vi "selectSurroundingPlatforms.vi"(9 "Number of surrounding\nplatforms to raise":i32=2, 11 "Start platform":i32) -> (2 "Platforms \nto raise":i32[](array[numeric]))   [LabVIEW 2017]
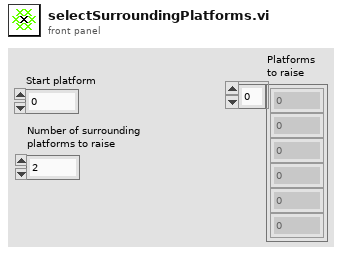
[diagram p1: front panel]
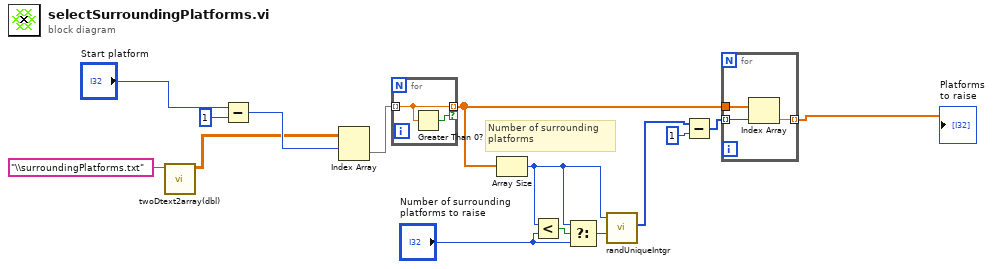
[diagram p0: block diagram]
diagram:
  # "Number of surrounding\nplatforms"
  n1 = call "twoDtext2array(dbl).vi"("String"="\\surroundingPlatforms.txt") -> ("all rows"=w1:dbl[][])  [unwired: 10 in]
  n2 = Subtract(x="Start platform", y=1) -> (x-y=w13:i32)
  n3 = Index Array(array=w1, index (row)=w13) -> (element=w12:dbl[])  [unwired: 1 in]
  n4 = for {
    tunnel: w12 -> [w17] mode=indexing
    tunnel: [w17] -> w11 mode=indexing if=w16
    n5 = Greater Than 0?(x=w17) -> (x > 0?=w16:bool)
  }
  n6 = Array Size(array=w11) -> (size(s)=w5:i32)
  n7 = Less?(x=w5, y="Number of surrounding\nplatforms to raise") -> (x < y?=w6:bool)
  n8 = Select(t=w5, s=w6, f="Number of surrounding\nplatforms to raise") -> (s? t:f=w3:i32)
  n9 = call "randUniqueIntgr.vi"("max rand number"=w5, "Number of Outputs"=w3) -> ("output"=w10:u32[])  [unwired: 8 in]
  n10 = Subtract(x=w10, y=1) -> (x-y=w8:u32[])
  n11 = for {
    tunnel: w8 -> [w19] mode=indexing
    tunnel: w11 -> [w20]
    tunnel: [w18] -> w2 mode=indexing
    n12 = Index Array(array=w20, index=w19) -> (element=w18:dbl)
  }
  "Platforms \nto raise" <- w2
